vi "OCR_Determine colors.vi"(8 "Error":errorcluster, 9 "Color Array":T1[](array[typedef]), 10 "Frame Type":T3, 11 "Border Color":u32(colorbox)) -> (0 "Error Out":errorcluster, 3 "Colors Out":T2)   [LabVIEW 2009]
uses:
  Controls/Enum/ENUM_Frame Template Select.ctl
  Controls/Cluster/Cluster_Icon Color Set.ctl
  Controls/Cluster/Cluster_Text Color Set.ctl
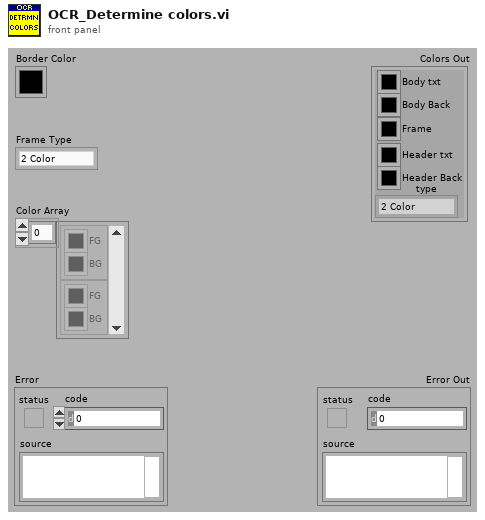
[diagram p1: front panel]
types:
  T1 = typedef "Cluster_Text Color Set.ctl" = cluster{"BG":u32, "FG":u32}
  T2 = typedef "Cluster_Icon Color Set.ctl" = cluster{"Body txt":u32, "Body Back":u32, "Frame":u32, "Header txt":u32, "Header Back":u32, "type":T3}
  T3 = typedef "ENUM_Frame Template Select.ctl" = enum16{"2 Color", "5 Color"}
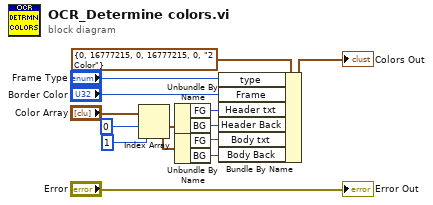
[diagram p0: block diagram]
diagram:
  n1 = Index Array(array="Color Array", index #1=0 ("index"), index #2=1 ("index")) -> (element #1=w4:T1, element #2=w3:T1)
  n2 = Unbundle By Name(w4) -> ("FG"=w10:u32, "BG"=w11:u32)
  n3 = Unbundle By Name(w3) -> ("FG"=w12:u32, "BG"=w13:u32)
  n4 = Bundle By Name(cluster=T2 {"Body txt"=0, "Body Back"=16777215, "Frame"=0, "Header txt"=16777215, "Header Back"=0, "type"=enum."2 Color"} ("Colors Out"), "type"="Frame Type", "Frame"="Border Color", "Header txt"=w10, "Header Back"=w11, "Body txt"=w12, "Body Back"=w13) -> (→"Colors Out":T2)
  "Error Out" <- "Error"
